vi "AUTOFLIM_Create_Filename.vi"(4 "Voltage":i32, 6 "X":dbl, 7 "Y":dbl, 8 "Term":string, 9 "Emitter #":i32, 10 "String":string, 11 "start path":path) -> (3 "appended path":path)   [LabVIEW 2023]
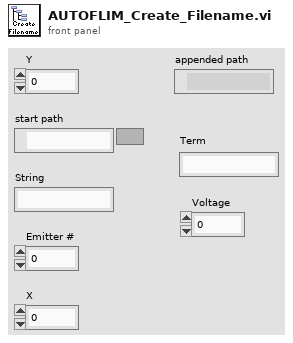
[diagram p1: front panel]
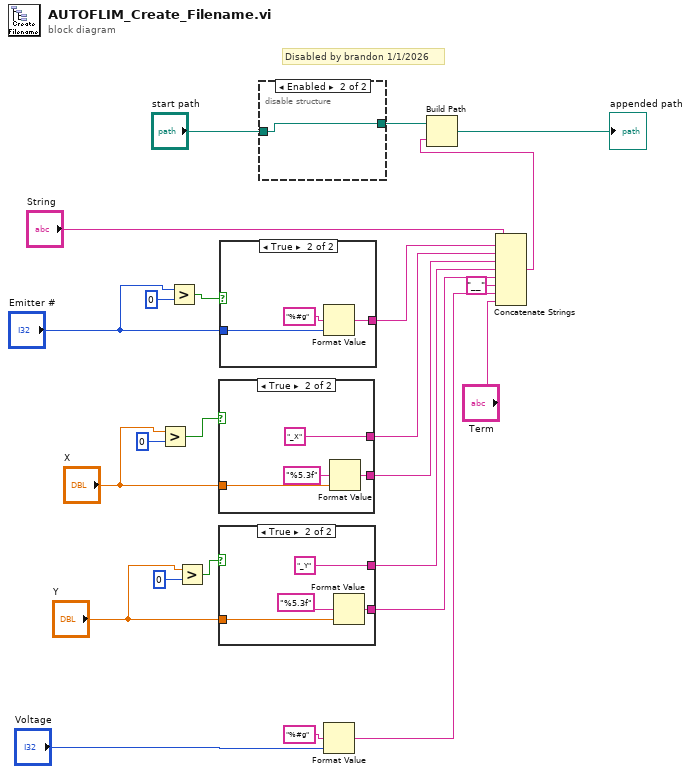
[diagram p0: block diagram]
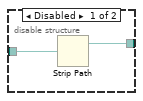
[diagram p2: hidden frame]
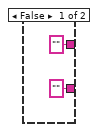
[diagram p3: hidden frame]
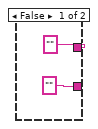
[diagram p4: hidden frame]
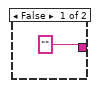
[diagram p5: hidden frame]
diagram:
  # "Disabled by brandon 1/1/2026"
  n1 = Greater?(x="X", y=0) -> (0:w11:bool)
  n2 = Greater?(x="Emitter #", y=0) -> (0:w15:bool)
  n3 = Greater?(x="Y", y=0) -> (0:w7:bool)
  n4 = case shown="True" w11 {
    tunnel: ["" ("output string") w30] -> w22
    tunnel: ["" "_X" ("string")] -> w21
    tunnel: "X" -> [_ w27]
    frame False {
    }
    frame True {
      n5 = Format Value(format string="%5.3f", value (0)=w27) -> (output string=w30:string)  [unwired: 1 in]
    }
  }
  n6 = case shown="True" w7 {
    tunnel: ["" ("output string") w36] -> w23
    tunnel: "Y" -> [_ w34]
    tunnel: ["" ("string") "_Y" ("string")] -> w9
    frame False {
    }
    frame True {
      n7 = Format Value(format string="%5.3f", value (0)=w34) -> (output string=w36:string)  [unwired: 1 in]
    }
  }
  n8 = case shown="True" w15 {
    tunnel: ["" w39] -> w20
    tunnel: "Emitter #" -> [_ w38]
    frame False {
    }
    frame True {
      n9 = Format Value(format string="%#g", value (0)=w38) -> (output string=w39:string)  [unwired: 1 in]
    }
  }
  n10 = disable-structure shown="Enabled" {
    disable-tunnel: "start path" -> [w42 w43]
    disable-tunnel: [w41 w43] -> w16
    frame Disabled {
      n11 = Strip Path(path=w42) -> (stripped path=w41:path)  [unwired: 1 out]
    }
    frame Enabled {
    }
  }
  n12 = Format Value(format string="%#g", value (0)="Voltage") -> (output string=w2:string)  [unwired: 1 in]
  n13 = Concatenate Strings("String", w20, w21, w22, w9, w23, "__" ("string"), w2, "Term") -> (w24:string)
  n14 = Build Path(base path=w16, name or relative path=w24) -> (appended path=→"appended path":path)
